vi "DegSinCos.vi"(3 "x":dbl[](array[numeric])) -> (0 "cos(x)":dbl[](array[numeric]), 1 "sin(x)":dbl[](array[numeric]))   [LabVIEW 2017]
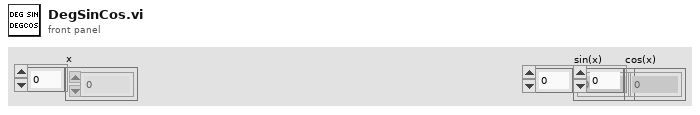
[diagram p1: front panel]
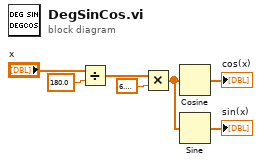
[diagram p0: block diagram]
diagram:
  n1 = Divide(x="x", y=180.0) -> (x/y=w7:dbl[])
  n2 = Multiply(x=w7, y=6.283185307179586) -> (x*y=w4:dbl[])
  n3 = Cosine(x=w4) -> (cos(x)=→"cos(x)":dbl[])
  n4 = Sine(x=w4) -> (sin(x)=→"sin(x)":dbl[])
